vi "Plot Editor.vi"(6 "Original Plot Idx":i32=-1, 7 "Original Graph Name":string, 8 "Error In":errorcluster, 9 "Plot Style in":T2={"Plot Index"=0, "Plot.Bar Plot Style"=0, "Plot.DigitalLineStyle"=1, "Plot.TransitionLocation"=2, "Plot.Transition Type"=0, "Plot.Fill To"=-1, "Plot.Fill/Pt. Color"=16777222, "Plot.Label Format"=3, "Plot.Line Style"=0, "Plot.Line Width"=1, "Plot.Plot Color"=16777222, "Plot.Plot Interpolation"=2, "Plot.Plot Name"="", "Plot.Point Style"=0, "Plot.Visible?"=TRUE, "Plot.XScaleIdx"=0, "Plot.YScaleIdx"=0, "Plot.Anti-aliased"=TRUE}, 10 "Plot in":T3, 11 "Original Graph Refnum":T1) -> (0 "Error Out":errorcluster, 1 "Plot Style out":T2, 2 "Plot out":T3)   [LabVIEW 2021, in "Plot Editor.lvlib"]
uses:
  Plot Editor.lvlib
  XY Graph/XY Graph Plot Properties.ctl
  XY Graph/XY Plot Data.ctl
  XY Graph/XY Graph Refnum.ctl
  Plot Editor Q [Element].ctl
  Plot Editor Q [Event] List.ctl
  Plot Editor Internal Variables.ctl
  XY Graph/XY Graph Event.ctl
  <vilib>/Utility/miscctls.llb/LVPoint32TypeDef.ctl
  <vilib>/Utility/error.llb/DialogType.ctl
  Variant/Variant to Data/Variant to String.vi
  Variant/Variant to Data/Variant to I32.vi
  XY Graph/XY Graph Add-Ons.lvlib
  GUI/GUI.lvlib
  Notebook/Notebook.lvlib
  Graphs.lvlib
  <userlib>/_OpenG.lib/string/string.llb/openg_string.lvlib
  Arrays/Define Ramp Array Dialog.vi
  Arrays/Arrays.lvlib
  Variant/Variant to Data/Variant to Data.lvlib
  Rich Text Box/Rich Text Box.lvlib
  Error/Error.lvlib
  Sound/Sound.lvlib
panel:
  out "Y Array Sum":dbl format="%#_5g"
  out "X Array Sum":dbl format="%#_5g"
  in  "X Array":dbl[](array[numeric])
  in  "Copy":bool
  in  "Cancel":bool
  out "Error":errorcluster
  in  "Reset Style":bool
  out "Y Array Size":i32 format="%#_5g"
  in  "Cancel Data Edit":bool
  in  "OK":bool
  out "X Array Size":i32 format="%#_5g"
  in  "Y Array":dbl[](array[numeric]) caption="X Array"
  out "Plot Preview":cluster{"X Array":dbl[], "Y Array":dbl[]}[](graph)
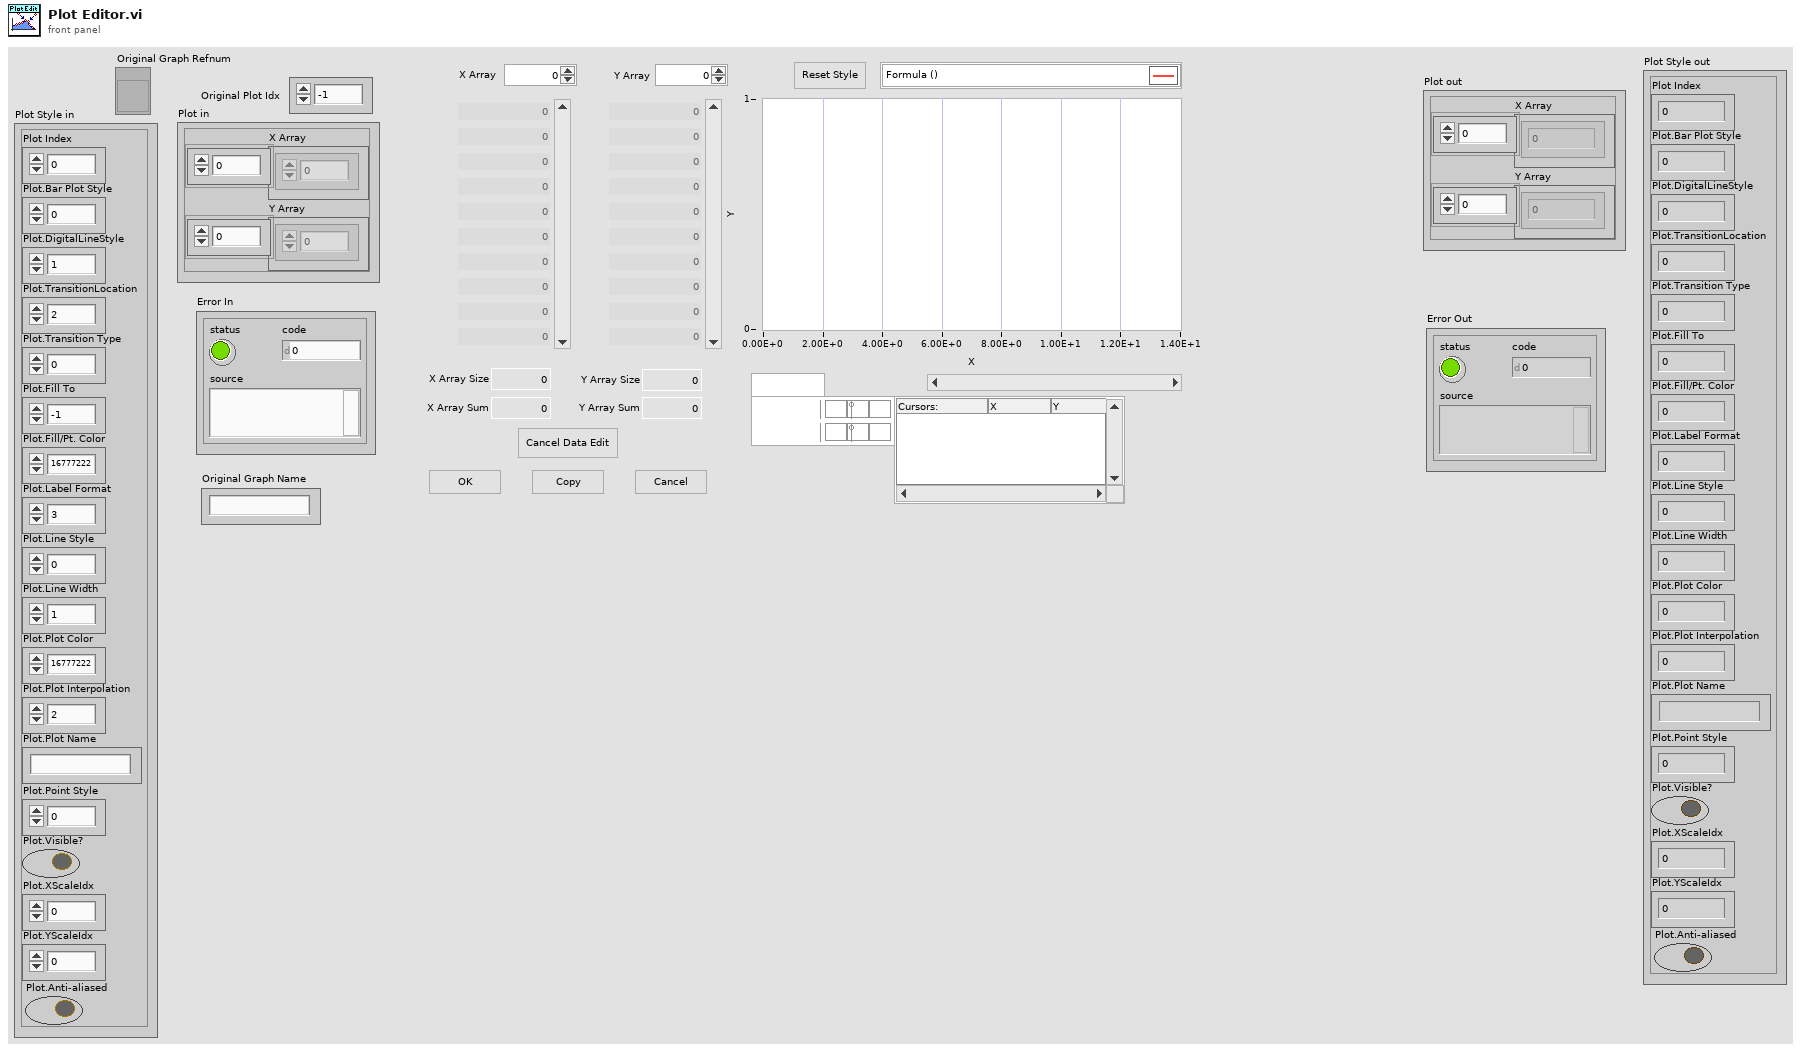
[diagram p1: front panel]
types:
  T1 = typedef "XY Graph Add-Ons.lvlib/XY Graph Refnum.ctl" = refnum<vi>
  T2 = typedef "XY Graph Add-Ons.lvlib/XY Graph Plot Properties.ctl" = cluster{"Plot Index":i32, "Plot.Bar Plot Style":u8, "Plot.DigitalLineStyle":u8, "Plot.TransitionLocation":u8, "Plot.Transition Type":u8, "Plot.Fill To":i16, "Plot.Fill/Pt. Color":u32, "Plot.Label Format":u8, "Plot.Line Style":u8, "Plot.Line Width":u8, "Plot.Plot Color":u32, "Plot.Plot Interpolation":u8, "Plot.Plot Name":string, "Plot.Point Style":u8, "Plot.Visible?":bool, "Plot.XScaleIdx":u32, "Plot.YScaleIdx":u32, "Plot.Anti-aliased":bool}
  T3 = typedef "XY Graph Add-Ons.lvlib/XY Plot Data.ctl" = cluster{"X Array":dbl[], "Y Array":dbl[]}
  T4 = typedef "Plot Editor.lvlib/Plot Editor Q [Element].ctl" = cluster{"Plot Editor Q Event":T5, "Data":variant}
  T5 = typedef "Plot Editor.lvlib/Plot Editor Q [Event] List.ctl" = enum16{"Idle", "Initialization", "Generic XY Graph Event", "Controls >> Store", "Store >> Plot", "Update Plot Style", "Check Data Array Alignment", "Reset Data", "Reset Style", "Accept & Quit", "Copy & Quit", "Save Plot", "Load Plot", "Delete out-of-bound Values", "Delete Element", "Insert Element Before", "Insert Element After", "Update output string", "Delete NaN-containing Pairs", "Delete Pairs with Duplicate X", "Fill Array with Ramp", "Quit"}
  T6 = typedef "Plot Editor.lvlib/Plot Editor Internal Variables.ctl" = cluster{"X Array":dbl[], "Y Array":dbl[], "XY Plot Properties":T2, "X Array Index Values":u32[], "Y Array Index Values":u32[], "Original XY Plot Properties":T2, "Original X Array":dbl[], "Original Y Array":dbl[], "VI title suffix":string, "Refnum based call":bool}
  T7 = typedef "XY Graph Add-Ons.lvlib/XY Graph Event.ctl" = cluster{"Item Tag":string, "XY Graph Refnum":refnum<vi>, "Coords":T8, "Item Path":string}
  T8 = typedef "LVPoint32TypeDef.ctl" = cluster{"Horizontal":i32, "Vertical":i32}
  T9 = typedef "Rich Text Box.lvlib/Text Formatting.ctl" = cluster{"Font":string, "Text Color":T10, "Text Background Color":T10, "Text Style":enum16{"Regular", "Bold", "Italic", "Underline", "Strikeout"}, "Font Size (Points)":dbl, "Text Alignment":i32}
  T10 = typedef "Rich Text Box.lvlib/Text Colors.ctl" = enum16{"Unchanged", "Black", "Blue", "Brown", "Gray", "Green", "Orange", "Pink", "Red", "White"}
  T11 = typedef "DialogType.ctl" = u16
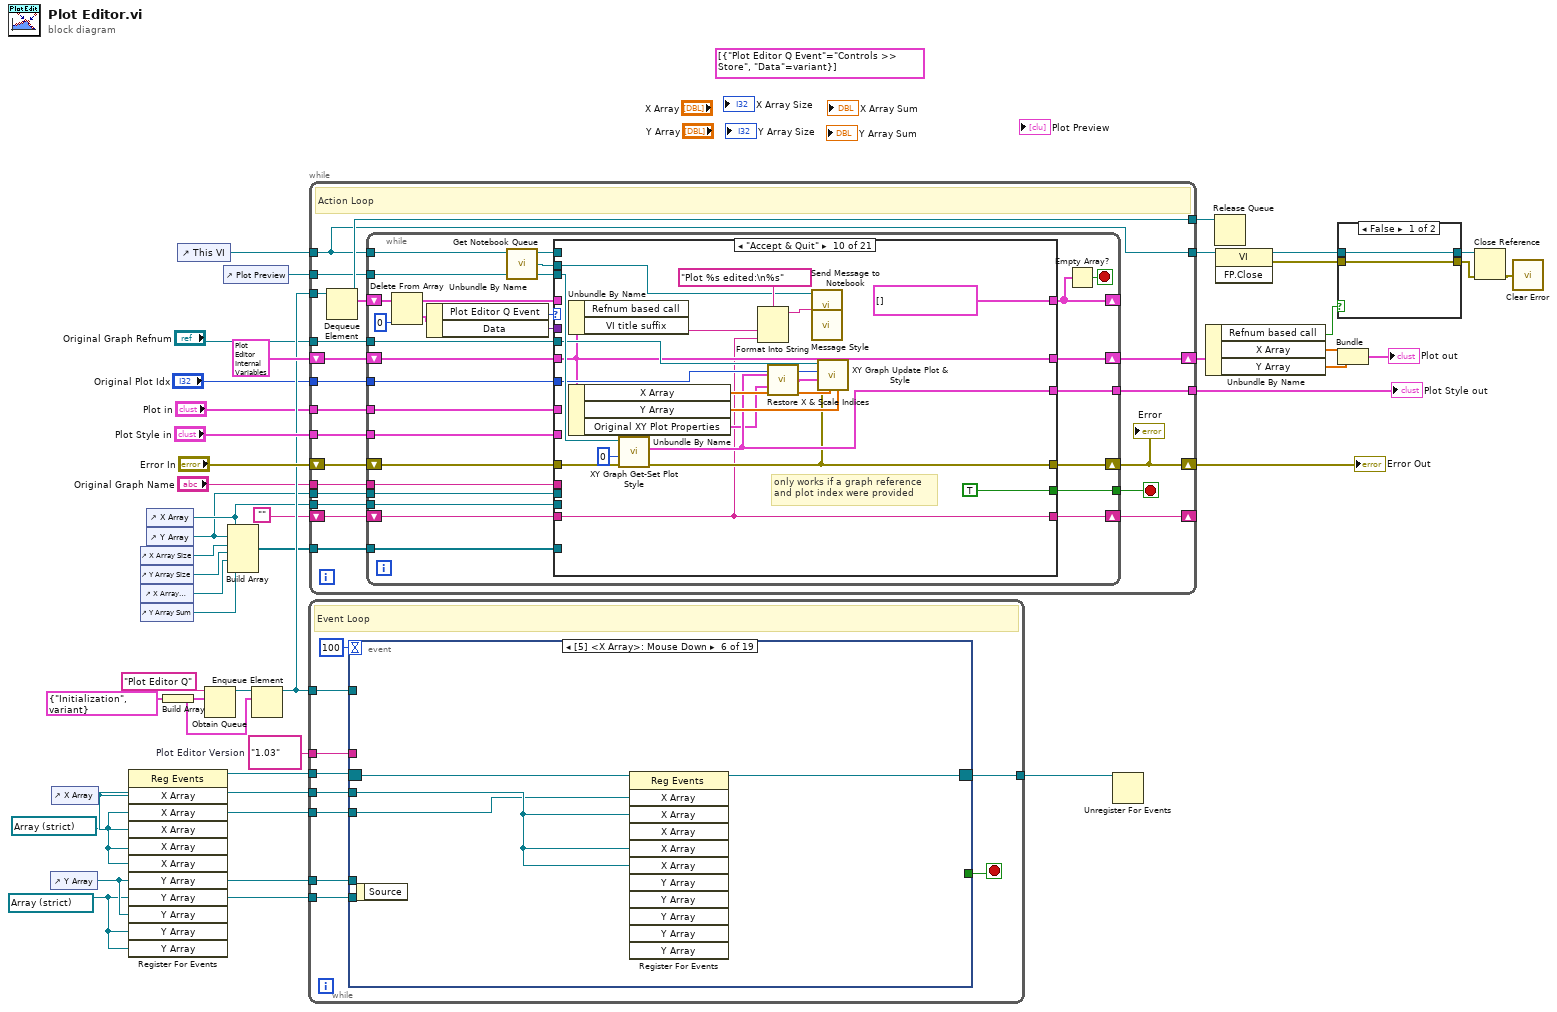
[diagram p0: block diagram]
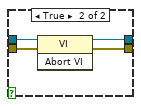
[diagram p2: hidden frame]
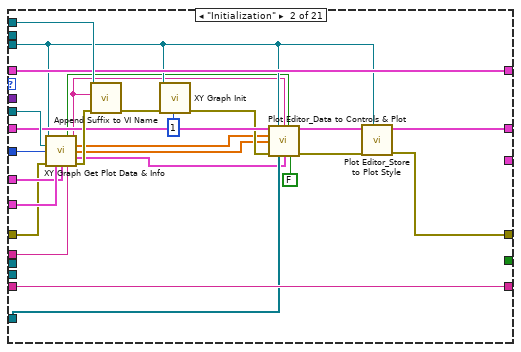
[diagram p4: hidden frame]
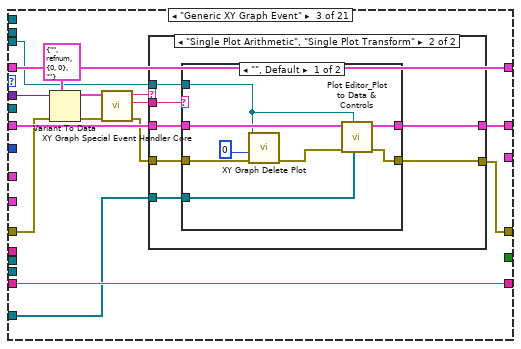
[diagram p5: hidden frame]
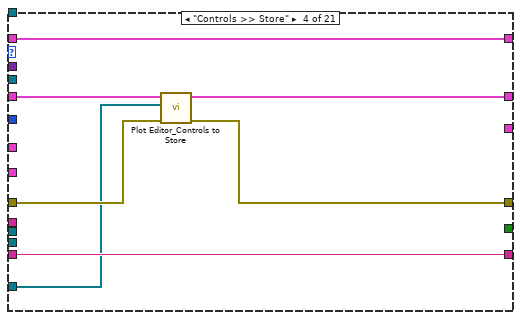
[diagram p8: hidden frame]
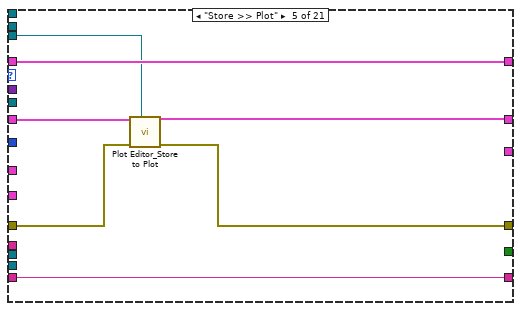
[diagram p9: hidden frame]
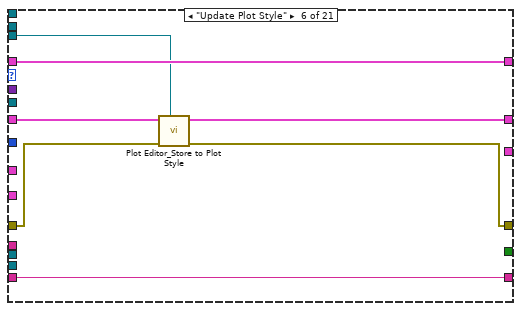
[diagram p10: hidden frame]
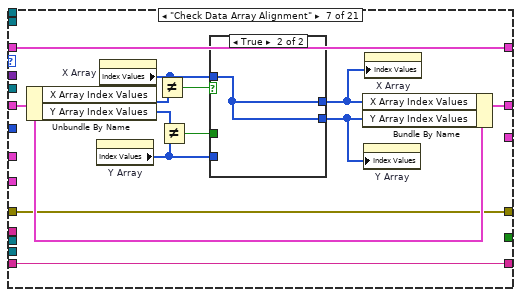
[diagram p11: hidden frame]
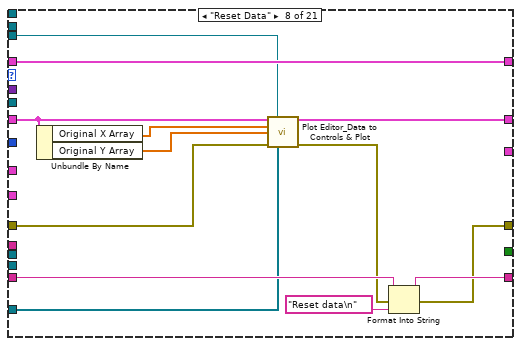
[diagram p14: hidden frame]
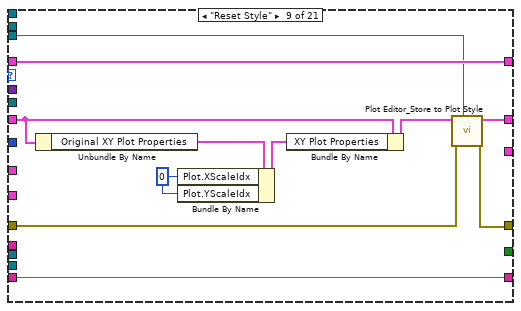
[diagram p15: hidden frame]
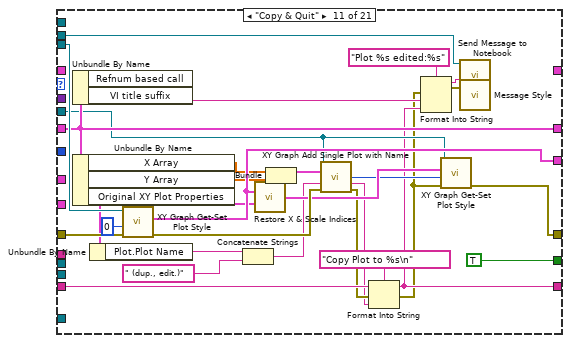
[diagram p16: hidden frame]
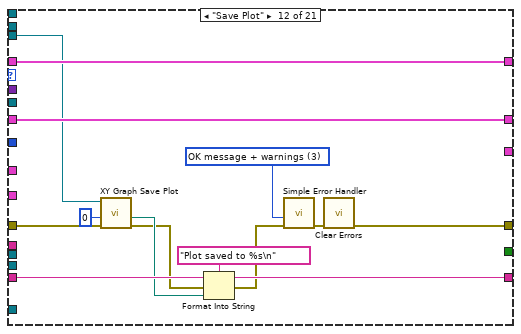
[diagram p17: hidden frame]
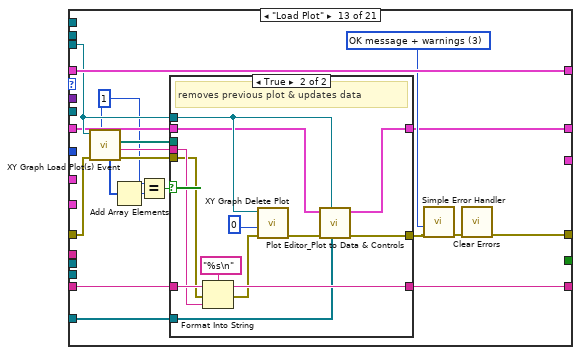
[diagram p18: hidden frame]
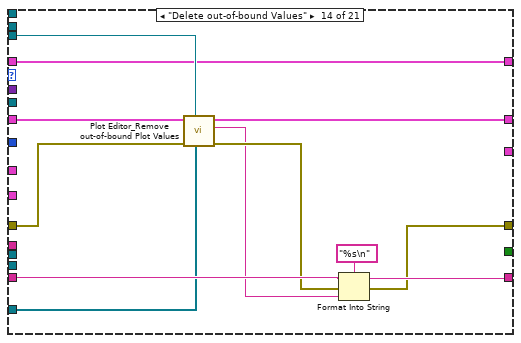
[diagram p20: hidden frame]
diagram:
  w4 = refnum<vi> refnum ("Y Array")
  w3 = refnum<vi> refnum ("X Array")
  (unwired) T4[] [{"Plot Editor Q Event"=enum."Controls >> Store", "Data"=variant}] ("array")
  w27 = "1.03"  # Plot Editor Version
  n1 = control-ref of="Y Array"() -> (w5:refnum<vi>)
  n2 = control-ref of="X Array"() -> (w6:refnum<vi>)
  n3 = register-events(w6, w3, w6, w3, w3, w5, w4, w5, w4, w4) -> (reference out=w26:refnum<event-registration>)  [unwired: 2 in, 1 out]
  n4 = control-ref of="X Array Size"() -> (w9:refnum<vi>)
  n5 = control-ref of="Y Array Size"() -> (w8:refnum<vi>)
  n6 = control-ref of="X Array Sum"() -> (w2:refnum<vi>)
  n7 = control-ref of="Y Array Sum"() -> (w1:refnum<vi>)
  n8 = control-ref of="X Array"() -> (w11:refnum<vi>)
  n9 = control-ref of="Y Array"() -> (w10:refnum<vi>)
  n10 = Build Array(T4 {"Plot Editor Q Event"=enum."Initialization", "Data"=variant} ("Plot Editor Q Element")) -> (w28:T4[])
  n11 = control-ref of="This VI"() -> (w18:refnum<vi>)
  n12 = Obtain Queue(name (unnamed)="Plot Editor Q", element data type=w28) -> (queue out=w41:refnum<queue>)  [unwired: 3 in, 2 out]
  n13 = control-ref of="Plot Preview"() -> (w36:refnum<vi>)
  n14 = Build Array(w11, w10, w9, w8, w2, w1) -> (w7:refnum<vi>[])
  n15 = Enqueue Element(queue=w41, element=w28) -> (queue out=w29:refnum<queue>)  [unwired: 2 in, 2 out]
  n16 = while {
    tunnel: w29 -> [w52]
    tunnel: w27 -> [w51]
    tunnel: w26 -> [w50]
    tunnel: w6 -> [w49]
    tunnel: w5 -> [w48]
    tunnel: [w47] -> w25
    tunnel: w3 -> [w46]
    tunnel: w4 -> [w45]
    stop <- w53 stop-if-true
    # "Event Loop"
    n17 = event shown="[5] <X Array>: Mouse Down" {
      selector: w50 -> [_ _ _ _ _ w179 w183 w186 w189 w195 w201 w205 w210 _ _ _ _ _ _]
      dyn-events: [_ _ _ _ _ w178 w182 w186 w189 w194 w200 w204 w209 _ _ _ _ _ _] -> w47
      timeout: 100 -> [_ _ _ _ _ _ _ _ _ _ _ _ _ _ _ _ _ _ _]
      tunnel: [w56 w58 _ _ _ _ _ _ _ _ _ _ _ _ _ _ TRUE ("Discard?") TRUE ("Discard?") TRUE ("Discard?")] -> w53
      tunnel: w52 -> [w55 w59 w102 w133 w160 _ _ w185 w188 w191 w196 _ _ w220 w222 w224 w227 w230 w233]
      tunnel: w51 -> [_ w57 _ _ _ _ _ _ _ _ _ _ _ _ _ _ _ _ _]
      tunnel: w49 -> [_ _ _ _ _ w177 _ _ _ w193 _ w203 w208 _ _ _ _ _ _]
      tunnel: w48 -> [_ _ _ _ _ _ w181 _ _ _ w198 _ w207 _ _ _ _ _ _]
      tunnel: w46 -> [_ _ _ _ _ w176 _ _ _ w192 _ w202 _ _ _ _ _ _ _]
      tunnel: w45 -> [_ _ _ _ _ _ w180 _ _ _ w199 _ w206 _ _ _ _ _ _]
      event Panel Close? {
        w56 = TRUE ("Discard?")
        n18 = event-data() -> ()  [unwired: 1 in, 1 out]
        n19 = Enqueue Element(queue=w55, element=T4[] [{"Plot Editor Q Event"=enum."Quit", "Data"=variant}]) -> ()  [unwired: 2 in, 3 out]
        n20 = event-data("Discard?"=w56) -> ()  [unwired: 1 in, 1 out]
      }
      event Menu Selection (User) {
        n21 = event-data() -> ("ItemTag"=w60:string)  [unwired: 1 in]
        n22 = case shown="\"Paste Data from Clipboard\"" w60 {
          tunnel: w59 -> [_ w62 w64 w68 w87 _]
          tunnel: [_ _ _ w65 _ _] -> w58
          tunnel: w57 -> [_ _ _ _ _ w95]
          frame "", Default {
          }
          frame "Save Plot" {
            n23 = Enqueue Element(queue=w62, element=T4[] [{"Plot Editor Q Event"=enum."Save Plot", "Data"=variant}]) -> ()  [unwired: 2 in, 3 out]
          }
          frame "Load Plot" {
            n24 = Enqueue Element(queue=w64, element=T4[] [{"Plot Editor Q Event"=enum."Load Plot", "Data"=variant}]) -> ()  [unwired: 2 in, 3 out]
          }
          frame "Quit" {
            n25 = call "Two Buttons Dialog Window with Resizeable Message.vi"("Message"="Are you sure you want to quit Plot Editor?\nQuitting will save the current changes and return to the original graph." ("message"), "OK Button Text"="Accept & Quit" ("T button name (\"OK\")")) -> ("OK?"=w65:bool)  [unwired: 7 in]
            n26 = case shown="True" w65 {
              tunnel: w68 -> [_ w70]
              frame False {
              }
              frame True {
                n27 = Enqueue Element(queue=w70, element=T4[] [{"Plot Editor Q Event"=enum."Accept & Quit", "Data"=variant}]) -> ()  [unwired: 2 in, 3 out]
              }
            }
          }
          frame "Paste Data from Clipboard" {
            w80 = "\n"
            n28 = invoke class="App" method="Clipboard.Read"() -> ("Read Clipbrd"=w76:string)  [unwired: 3 in, 2 out]
            n29 = call <userlib>:"String to 1D Array__ogtk.vi"("delimiter (Tab)"=w80, "string"=w76) -> ("Array of Strings"=w85:string[])  [unwired: 9 in]
            n30 = Delete From Array(array=w85, length=1, index=0) -> (array with subset deleted=w82:string[])  [unwired: 1 out]
            n31 = call <userlib>:"1D Array to String__ogtk.vi"("delimiter (Tab)"=w80, "Array of Strings"=w82) -> ("delimited string"=w81:string)  [unwired: 9 in]
            n32 = Spreadsheet String To Array(format string="%#g", spreadsheet string=w81) -> (array=w88:dbl[][])  [unwired: 2 in]
            n33 = Transpose 2D Array(2D array=w88) -> (transposed array=w79:dbl[][])
            n34 = Index Array(array=w79) -> (element #1=w72:dbl[], element #2=w71:dbl[])  [unwired: 4 in]
            n35 = Array Size(array=w72) -> (size(s)=w78:i32)
            n36 = Array Size(array=w71) -> (size(s)=w77:i32)
            n37 = Empty Array?(array=w72) -> (empty?=w75:bool)
            n38 = Not Equal?(x=w78, y=w77) -> (x != y?=w74:bool)
            n39 = Or(x=w75, y=w74) -> (x .or. y?=w73:bool)
            n40 = case shown="True" w73 {
              tunnel: w87 -> [w92 _]
              tunnel: w72 -> [w90 _]
              tunnel: w71 -> [w89 _]
              frame False {
                n41 = local write "X Array"(w90) -> ()
                n42 = local write "Y Array"(w89) -> ()
                n43 = Enqueue Element(queue=w92, element=T4[] [{"Plot Editor Q Event"=enum."Controls >> Store", "Data"=variant}, {"Plot Editor Q Event"=enum."Store >> Plot", "Data"=variant}]) -> ()  [unwired: 2 in, 3 out]
              }
              frame True {
                n44 = One Button Dialog(message="The clipboard doesn't contain any valid plot data...") -> ()  [unwired: 1 in, 1 out]
                n45 = call "Play Error Sound.vi"() -> ()  [unwired: 27 in, 1 out]
              }
            }
          }
          frame "About..." {
            n46 = Format Into String(format string="                                      Plot Editor\n                                      version %s\n\n                              Author: X. Michalet\n(c) 2017-2022 The Regents of the  University of California" ("message"), w95) -> (resulting string=w94:string)  [unwired: 2 in, 1 out]
            n47 = One Button Dialog(message=w94) -> ()  [unwired: 1 in, 1 out]
          }
        }
      }
      event "X Array": Shortcut Menu Selection (User) {
        n48 = event-data() -> ("ItemTag"=w103:string, "CtlRef"=w100:refnum<vi>, "Coords"=w99:T8)  [unwired: 1 in]
        n49 = case shown="\"Delete NaN-containing Pairs\"" w103 {
          tunnel: [w104 w110 w116 w122 w125 w127] -> w101
          tunnel: w100 -> [_ w109 w115 w121 _ _]
          tunnel: w99 -> [_ w108 w114 w120 _ _]
          frame "", Default {
            n50 = Build Array(T4 {"Plot Editor Q Event"=enum."Idle", "Data"=variant} ("Plot Editor Q Element")) -> (w104:T4[])
          }
          frame "Delete Element" {
            n51 = Bundle("CtlRef"=w109, "Coords"=w108) -> (w106:cluster{"CtlRef":refnum<vi>, "Coords":T8})  [unwired: 1 in]
            n52 = Bundle By Name(cluster=T4 {"Plot Editor Q Event"=enum."Delete Element", "Data"=variant} ("Plot Editor Q Element"), "Data"=w106) -> (w107:T4)
            n53 = Build Array(w107) -> (w110:T4[])
          }
          frame "Insert Element Before" {
            n54 = Bundle("CtlRef"=w115, "Coords"=w114) -> (w112:cluster{"CtlRef":refnum<vi>, "Coords":T8})  [unwired: 1 in]
            n55 = Bundle By Name(cluster=T4 {"Plot Editor Q Event"=enum."Insert Element Before", "Data"=variant} ("Plot Editor Q Element"), "Data"=w112) -> (w113:T4)
            n56 = Build Array(w113) -> (w116:T4[])
          }
          frame "Insert Element After" {
            n57 = Bundle("CtlRef"=w121, "Coords"=w120) -> (w118:cluster{"CtlRef":refnum<vi>, "Coords":T8})  [unwired: 1 in]
            n58 = Bundle By Name(cluster=T4 {"Plot Editor Q Event"=enum."Insert Element After", "Data"=variant} ("Plot Editor Q Element"), "Data"=w118) -> (w119:T4)
            n59 = Build Array(w119) -> (w122:T4[])
          }
          frame "Fill Array with Ramp" {
            n60 = Build Array(T4 {"Plot Editor Q Event"=enum."Fill Array with Ramp", "Data"=variant} ("Plot Editor Q Element")) -> (w125:T4[])
          }
          frame "Delete NaN-containing Pairs" {
            n61 = Build Array(T4 {"Plot Editor Q Event"=enum."Delete NaN-containing Pairs", "Data"=variant} ("Plot Editor Q Element")) -> (w127:T4[])
          }
        }
        n62 = Build Array (concatenate)(w101, T4[] [{"Plot Editor Q Event"=enum."Controls >> Store", "Data"=variant}, {"Plot Editor Q Event"=enum."Store >> Plot", "Data"=variant}] ("array")) -> (w98:T4[])
        n63 = Enqueue Element(queue=w102, element=w98) -> ()  [unwired: 2 in, 3 out]
      }
      event "Y Array": Shortcut Menu Selection (User) {
        n64 = event-data() -> ("ItemTag"=w134:string, "CtlRef"=w132:refnum<vi>, "Coords"=w131:T8)  [unwired: 1 in]
        n65 = case shown="\"Remove NaN-containing Pairs\"" w134 {
          tunnel: [w135 w139 w145 w151 w156] -> w130
          tunnel: w132 -> [_ w138 w144 w150 _]
          tunnel: w131 -> [_ w137 w143 w149 _]
          frame "", Default {
            n66 = Build Array(T4 {"Plot Editor Q Event"=enum."Idle", "Data"=variant} ("Plot Editor Q Element")) -> (w135:T4[])
          }
          frame "Delete Element" {
            n67 = Bundle("CtlRef"=w138, "Coords"=w137) -> (w141:cluster{"CtlRef":refnum<vi>, "Coords":T8})  [unwired: 1 in]
            n68 = Bundle By Name(cluster=T4 {"Plot Editor Q Event"=enum."Delete Element", "Data"=variant} ("Plot Editor Q Element"), "Data"=w141) -> (w142:T4)
            n69 = Build Array(w142) -> (w139:T4[])
          }
          frame "Insert Element Before" {
            n70 = Bundle("CtlRef"=w144, "Coords"=w143) -> (w147:cluster{"CtlRef":refnum<vi>, "Coords":T8})  [unwired: 1 in]
            n71 = Bundle By Name(cluster=T4 {"Plot Editor Q Event"=enum."Insert Element Before", "Data"=variant} ("Plot Editor Q Element"), "Data"=w147) -> (w148:T4)
            n72 = Build Array(w148) -> (w145:T4[])
          }
          frame "Insert Element After" {
            n73 = Bundle("CtlRef"=w150, "Coords"=w149) -> (w153:cluster{"CtlRef":refnum<vi>, "Coords":T8})  [unwired: 1 in]
            n74 = Bundle By Name(cluster=T4 {"Plot Editor Q Event"=enum."Insert Element After", "Data"=variant} ("Plot Editor Q Element"), "Data"=w153) -> (w154:T4)
            n75 = Build Array(w154) -> (w151:T4[])
          }
          frame "Remove NaN-containing Pairs" {
            n76 = Build Array(T4 {"Plot Editor Q Event"=enum."Delete NaN-containing Pairs", "Data"=variant} ("Plot Editor Q Element")) -> (w156:T4[])
          }
        }
        n77 = Build Array (concatenate)(w130, T4[] [{"Plot Editor Q Event"=enum."Controls >> Store", "Data"=variant}, {"Plot Editor Q Event"=enum."Store >> Plot", "Data"=variant}] ("array")) -> (w129:T4[])
        n78 = Enqueue Element(queue=w133, element=w129) -> ()  [unwired: 2 in, 3 out]
      }
      event "Plot Preview": Shortcut Menu Selection (User) {
        n79 = event-data() -> ("ItemTag"=w161:string, "CtlRef"=w159:refnum<vi>, "Coords"=w158:T8, "ItemPath"=w157:string)  [unwired: 1 in]
        n80 = case shown="\"Load Plot\"" w161 {
          selector: w161 -> [w170 _ _]
          tunnel: w160 -> [w166 w173 w175]
          tunnel: w159 -> [w169 _ _]
          tunnel: w158 -> [w168 _ _]
          tunnel: w157 -> [w167 _ _]
          frame "", Default {
            n81 = Bundle By Name(cluster=T7 {"Item Tag"="", "XY Graph Refnum"=refnum, "Coords"={"Horizontal"=0, "Vertical"=0}, "Item Path"=""} ("XY Graph Event"), "Item Tag"=w170, "XY Graph Refnum"=w169, "Coords"=w168, "Item Path"=w167) -> (w163:T7)
            n82 = Bundle By Name(cluster=T4 {"Plot Editor Q Event"=enum."Generic XY Graph Event", "Data"=variant} ("element"), "Data"=w163) -> (w164:T4)
            n83 = Build Array(w164) -> (w162:T4[])
            n84 = Enqueue Element(queue=w166, element=w162) -> ()  [unwired: 2 in, 3 out]
          }
          frame "Load Plot" {
            n85 = Enqueue Element(queue=w173, element=T4[] [{"Plot Editor Q Event"=enum."Load Plot", "Data"=variant}]) -> ()  [unwired: 2 in, 3 out]
          }
          frame "Delete out-of-bound Values" {
            n86 = Enqueue Element(queue=w175, element=T4[] [{"Plot Editor Q Event"=enum."Delete out-of-bound Values", "Data"=variant}]) -> ()  [unwired: 2 in, 3 out]
          }
        }
      }
      event Mouse Down {
        n87 = event-data() -> ()  [unwired: 1 in, 1 out]
        n88 = register-events(reference=w179, w176, w177, w177, w177) -> (reference out=w178:refnum<event-registration>)  [unwired: 7 in, 1 out]
      }
      event Mouse Down {
        n89 = event-data() -> ()  [unwired: 1 in, 1 out]
        n90 = register-events(reference=w183, w180, w181, w181, w181) -> (reference out=w182:refnum<event-registration>)  [unwired: 7 in, 1 out]
      }
      event Mouse Move; Mouse Wheel {
        n91 = event-data() -> ()  [unwired: 1 in, 1 out]
        n92 = Enqueue Element(queue=w185, element=T4[] [{"Plot Editor Q Event"=enum."Check Data Array Alignment", "Data"=variant}]) -> ()  [unwired: 2 in, 3 out]
      }
      event Timeout {
        n93 = event-data() -> ()  [unwired: 1 in, 1 out]
        n94 = Enqueue Element(queue=w188, element=T4[] [{"Plot Editor Q Event"=enum."Check Data Array Alignment", "Data"=variant}]) -> ()  [unwired: 2 in, 3 out]
      }
      event Mouse Up {
        n95 = event-data() -> ()  [unwired: 1 in, 1 out]
        n96 = register-events(reference=w195, w193, w192, w192) -> (reference out=w194:refnum<event-registration>)  [unwired: 8 in, 1 out]
        n97 = Enqueue Element(queue=w191, element=T4[] [{"Plot Editor Q Event"=enum."Check Data Array Alignment", "Data"=variant}]) -> ()  [unwired: 2 in, 3 out]
      }
      event Mouse Up {
        n98 = event-data() -> ()  [unwired: 1 in, 1 out]
        n99 = register-events(reference=w201, w198, w199, w199) -> (reference out=w200:refnum<event-registration>)  [unwired: 8 in, 1 out]
        n100 = Enqueue Element(queue=w196, element=T4[] [{"Plot Editor Q Event"=enum."Check Data Array Alignment", "Data"=variant}]) -> ()  [unwired: 2 in, 3 out]
      }
      event Mouse Leave {
        n101 = event-data() -> ()  [unwired: 1 in, 1 out]
        n102 = register-events(reference=w205, w203, w202, w202, w202) -> (reference out=w204:refnum<event-registration>)  [unwired: 7 in, 1 out]
      }
      event Mouse Leave {
        n103 = event-data() -> ()  [unwired: 1 in, 1 out]
        n104 = register-events(reference=w210, w208, w207, w206, w206, w206) -> (reference out=w209:refnum<event-registration>)  [unwired: 6 in, 1 out]
      }
      event "X Array", "Y Array": Value Change {
        n105 = event-data() -> ("CtlRef"=w215:refnum<vi>)  [unwired: 1 in]
        n106 = property class="Arr (strict)"(reference=w215) -> (error out=w212:errorcluster, "Label.Text"=w213:string)  [unwired: 1 in, 1 out]
        n107 = Format Into String(format string="User added %s data", error in=w212, w213) -> (resulting string=w211:string)  [unwired: 1 in, 1 out]
        n108 = Bundle By Name(cluster=T4 {"Plot Editor Q Event"=enum."Update output string", "Data"=variant} ("Plot Editor Q Element"), "Data"=w211) -> (w216:T4)
        n109 = Build Array (concatenate)(T4[] [{"Plot Editor Q Event"=enum."Controls >> Store", "Data"=variant}, {"Plot Editor Q Event"=enum."Store >> Plot", "Data"=variant}, {"Plot Editor Q Event"=enum."Check Data Array Alignment", "Data"=variant}] ("element"), w216) -> (w218:T4[])
        n110 = Enqueue Element(queue=w220, element=w218) -> ()  [unwired: 2 in, 3 out]
      }
      event "Reset Style": Value Change {
        n111 = event-data() -> ()  [unwired: 1 in, 1 out]
        n112 = Enqueue Element(queue=w222, element=T4[] [{"Plot Editor Q Event"=enum."Reset Style", "Data"=variant}]) -> ()  [unwired: 2 in, 3 out]
      }
      event "Cancel Data Edit": Value Change {
        n113 = event-data() -> ()  [unwired: 1 in, 1 out]
        n114 = Enqueue Element(queue=w224, element=T4[] [{"Plot Editor Q Event"=enum."Reset Data", "Data"=variant}]) -> ()  [unwired: 2 in, 3 out]
      }
      event "OK": Value Change {
        n115 = event-data() -> ()  [unwired: 1 in, 1 out]
        n116 = Enqueue Element(queue=w227, element=T4[] [{"Plot Editor Q Event"=enum."Accept & Quit", "Data"=variant}]) -> ()  [unwired: 2 in, 3 out]
      }
      event "Copy": Value Change {
        n117 = event-data() -> ()  [unwired: 1 in, 1 out]
        n118 = Enqueue Element(queue=w230, element=T4[] [{"Plot Editor Q Event"=enum."Copy & Quit", "Data"=variant}]) -> ()  [unwired: 2 in, 3 out]
      }
      event "Cancel": Value Change {
        n119 = event-data() -> ()  [unwired: 1 in, 1 out]
        n120 = Enqueue Element(queue=w233, element=T4[] [{"Plot Editor Q Event"=enum."Quit", "Data"=variant}]) -> ()  [unwired: 2 in, 3 out]
      }
    }
  }
  n121 = while {
    tunnel: w29 -> [w254]
    tunnel: [w251] -> w40
    shift-right: [w248] -> w34
    shift-left: T6 {"X Array"=[], "Y Array"=[], "XY Plot Properties"={"Plot Index"=0, "Plot.Bar Plot Style"=0, "Plot.DigitalLineStyle"=0, "Plot.TransitionLocation"=0, "Plot.Transition Type"=0, "Plot.Fill To"=-1, "Plot.Fill/Pt. Color"=0, "Plot.Label Format"=0, "Plot.Line Style"=0, "Plot.Line Width"=0, "Plot.Plot Color"=0, "Plot.Plot Interpolation"=0, "Plot.Plot Name"="Plot", "Plot.Point Style"=0, "Plot.Visible?"=FALSE, "Plot.XScaleIdx"=0, "Plot.YScaleIdx"=0, "Plot.Anti-aliased"=FALSE}, "X Array Index Values"=[], "Y Array Index Values"=[], "Original XY Plot Properties"={"Plot Index"=0, "Plot.Bar Plot Style"=0, "Plot.DigitalLineStyle"=0, "Plot.TransitionLocation"=0, "Plot.Transition Type"=0, "Plot.Fill To"=0, "Plot.Fill/Pt. Color"=0, "Plot.Label Format"=0, "Plot.Line Style"=0, "Plot.Line Width"=0, "Plot.Plot Color"=0, "Plot.Plot Interpolation"=0, "Plot.Plot Name"="", "Plot.Point Style"=0, "Plot.Visible?"=FALSE, "Plot.XScaleIdx"=0, "Plot.YScaleIdx"=0, "Plot.Anti-aliased"=FALSE}, "Original X Array"=[], "Original Y Array"=[], "VI title suffix"="", "Refnum based call"=FALSE} ("Plot Editor Internal Data") -> [w250]
    shift-right: [w239] -> w35
    shift-left: "Error In" -> [w247]
    tunnel: "Plot Style in" -> [w249]
    tunnel: w36 -> [w246]
    tunnel: [w245] -> w30
    tunnel: "Original Graph Refnum" -> [w244]
    tunnel: "Original Plot Idx" -> [w243]
    tunnel: "Plot in" -> [w242]
    tunnel: "Original Graph Name" -> [w241]
    tunnel: w18 -> [w240]
    tunnel: [w240] -> w20
    shift-right: [w237] -> _
    shift-left: "" -> [w238]
    tunnel: w11 -> [w236]
    tunnel: w10 -> [w235]
    tunnel: w7 -> [w234]
    stop <- w252 stop-if-true
    # "Action Loop"
    n122 = Dequeue Element(queue=w254) -> (queue out=w251:refnum<queue>, element=w253:T4[])  [unwired: 2 in, 2 out]
    n123 = while {
      tunnel: [w281] -> w252
      shift-right: [w277] -> _
      shift-left: w253 -> [w280]
      tunnel: w249 -> [w274]
      tunnel: w246 -> [w256]
      shift-right: [w273] -> w248
      shift-left: w250 -> [w275]
      shift-right: [w269] -> w239
      shift-left: w247 -> [w270]
      tunnel: [w268] -> w245
      tunnel: w244 -> [w267]
      tunnel: w243 -> [w266]
      tunnel: w242 -> [w265]
      tunnel: w241 -> [w264]
      tunnel: w240 -> [w263]
      shift-right: [w260] -> w237
      shift-left: w238 -> [w261]
      tunnel: w236 -> [w259]
      tunnel: w235 -> [w258]
      tunnel: w234 -> [w257]
      stop <- w276 stop-if-true
      n124 = Delete From Array(array=w280, index=0) -> (deleted portion=w272:T4, array with subset deleted=w278:T4[])  [unwired: 1 in]
      n125 = Unbundle By Name(w272) -> ("Plot Editor Q Event"=w271:T5, "Data"=w262:variant)
      n126 = call "Get Notebook Queue.vi"() -> ("Notebook Queue"=w255:refnum<queue>)  [unwired: 9 in]
      n127 = case shown="\"Accept & Quit\"" w271 {
        tunnel: [_ _ _ _ _ _ _ _ _ TRUE TRUE _ _ _ _ _ _ _ _ _ TRUE] -> w281
        tunnel: w278 -> [w285 w300 w326 w352 w359 w366 w373 w398 w412 _ _ w476 w495 w515 w531 w576 w621 w668 w673 w706 _]
        tunnel: [w285 w300 w326 w352 w359 w366 w373 w398 w412 T4[] [] _ w476 w495 w515 w530 w575 w620 w668 w673 w703 T4[] []] -> w277
        tunnel: w275 -> [w283 w297 w320 w350 w355 w362 w375 w395 w411 w425 w460 w475 w485 w514 w527 w572 w617 w660 w672 w713 w742]
        tunnel: w274 -> [_ w309 _ _ _ _ _ _ _ _ _ _ _ _ _ _ _ _ _ _ _]
        tunnel: [w283 w298 w319 w349 w356 w361 w374 w394 w405 w425 w460 w475 w484 w513 w524 w571 w616 w660 w670 w712 w743] -> w273
        tunnel: w270 -> [w284 w307 w316 w347 w353 w365 w370 w393 w404 w423 w458 w473 w494 w523 w528 w574 w619 w662 w678 w711 _]
        tunnel: [w284 w299 w317 w348 w354 w364 w370 w397 w403 w421 w454 w470 w491 w518 w529 w573 w618 w663 w676 w704 _] -> w269
        tunnel: [_ _ _ _ _ _ _ _ _ w422 w457 _ _ _ _ _ _ _ _ _ w739] -> w268
        tunnel: w267 -> [_ w311 _ _ _ _ _ _ _ w429 w453 _ _ _ _ _ _ _ _ _ _]
        tunnel: w266 -> [_ w310 _ _ _ _ _ _ _ w428 _ _ _ _ _ _ _ _ _ _ _]
        tunnel: w265 -> [_ w308 _ _ _ _ _ _ _ _ _ _ _ _ _ _ _ _ _ _ _]
        tunnel: w264 -> [_ w306 _ _ _ _ _ _ _ _ _ _ _ _ _ _ _ _ _ _ _]
        tunnel: w263 -> [_ w305 _ _ _ _ _ _ _ _ _ _ _ _ _ _ _ _ _ _ _]
        tunnel: w262 -> [_ _ w321 _ _ _ _ _ _ _ _ _ _ _ w543 w588 w633 w667 w684 _ _]
        tunnel: w259 -> [_ _ _ _ _ _ _ _ _ _ _ _ _ _ w537 w582 w630 _ _ _ _]
        tunnel: w258 -> [_ _ _ _ _ _ _ _ _ _ _ _ _ _ w536 w581 w629 _ _ _ _]
        tunnel: w261 -> [w282 w302 w325 w351 w358 w363 w369 w401 w407 w414 w443 w468 w483 w522 w533 w578 w623 w666 w680 w708 w737]
        tunnel: [w282 w302 w325 w351 w358 w363 w369 w400 w407 w414 w437 w465 w482 w521 w532 w577 w622 w665 w679 w707 w737] -> w260
        tunnel: w257 -> [_ w292 w313 w346 _ _ _ w389 _ _ _ _ w479 w512 w526 w569 w615 _ w671 w702 _]
        tunnel: w256 -> [_ w295 w314 _ w357 w360 _ w390 w402 w431 w462 w474 w487 w517 w525 w570 w614 _ w669 w701 _]
        tunnel: w255 -> [_ _ _ _ _ _ _ _ _ w413 w433 _ _ _ _ _ _ _ _ _ _]
        frame "Idle" {
        }
        frame "Initialization" {
          n128 = call "XY Graph Get Plot Data & Info.vi"("Destination Graph"=w295, "Original Graph"=w311, "Original Plot Idx"=w310, "Error In"=w307, "Plot Style in"=w309, "Plot in"=w308, "Graph Origin Name"=w306) -> ("Refnum based call"=w286:bool, "VI Title Suffix"=w287:string, "X Array"=w291:dbl[], "Y Array"=w290:dbl[], "Plot Style out"=w288:T2, "Error Out"=w304:errorcluster)  [unwired: 3 in]
          n129 = call "Append Suffix to VI Name.vi"("error in (no error)"=w304, "VI Title Suffix"=w287, "VI in"=w305) -> ("Error Out"=w301:errorcluster)  [unwired: 8 in]
          n130 = call "XY Graph Init.vi"("Max Legend Size (8)"=1 ("Plot.XScaleIdx"), "Error In"=w301, "XYGraph in"=w295) -> ("Error Out"=w294:errorcluster)  [unwired: 8 in]
          n131 = call "Plot Editor_Data to Controls & Plot.vi"("Plot Editor Internal Data"=w297, "XYGraph in"=w295, "VI Title Suffix"=w287, "Refnum based call"=w286, "X Array"=w291, "Y Array"=w290, "error in (no error)"=w294, "Control Refnums"=w292, "Plot Style"=w288, "Data only (T)"=FALSE) -> ("Plot Editor Internal Data"=w296:T6, "error out"=w293:errorcluster)  [unwired: 4 in]
          n132 = call "Plot Editor_Store to Plot Style.vi"("XYGraph in"=w295, "error in (no error)"=w293, "Plot Editor Internal Data"=w296) -> ("error out"=w299:errorcluster, "Plot Editor Internal Data (dup)"=w298:T6)  [unwired: 7 in]
        }
        frame "Generic XY Graph Event" {
          n133 = Variant To Data(error in=w316, type=T7 {"Item Tag"="", "XY Graph Refnum"=refnum, "Coords"={"Horizontal"=0, "Vertical"=0}, "Item Path"=""} ("XY Graph Event"), Variant=w321) -> (data=w322:T7, error out=w323:errorcluster)
          n134 = call "XY Graph Special Event Handler Core.vi"("error in (no error)"=w323, "XY Graph Event"=w322) -> ("error out"=w318:errorcluster, "Message"=w312:string, "Menu Item Tag (dup)"=w315:string)  [unwired: 5 in, 2 out]
          n135 = case shown="\"Single Plot Arithmetic\", \"Single Plot Transform\"" w315 {
            tunnel: w320 -> [w328 w335]
            tunnel: [w328 w332] -> w319
            tunnel: w318 -> [w327 w334]
            tunnel: [w327 w331] -> w317
            tunnel: w314 -> [_ w333]
            tunnel: w313 -> [_ w330]
            tunnel: w312 -> [_ w329]
            frame "", Default {
            }
            frame "Single Plot Arithmetic", "Single Plot Transform" {
              n136 = case shown="\"\", Default" w329 {
                tunnel: w335 -> [w342 w345]
                tunnel: w334 -> [w341 w344]
                tunnel: w333 -> [w339 _]
                tunnel: [w338 w345] -> w332
                tunnel: [w337 w344] -> w331
                tunnel: w330 -> [w336 _]
                frame "", Default {
                  n137 = call "XY Graph Delete Plot.vi"("Error In"=w341, "Plot Index"=0, "XYGraph Ref"=w339) -> ("Error Out"=w340:errorcluster)  [unwired: 5 in, 3 out]
                  n138 = call "Plot Editor_Plot to Data & Controls.vi"("Control Refnums"=w336, "XYGraph in"=w339, "error in (no error)"=w340, "Plot Editor Internal Data in"=w342) -> ("error out"=w337:errorcluster, "Plot Editor Internal Data out"=w338:T6)  [unwired: 6 in]
                }
                frame "Operation cancelled by user." {
                }
              }
            }
          }
        }
        frame "Controls >> Store" {
          n139 = call "Plot Editor_Controls to Store.vi"("Error In"=w347, "Control Refnums"=w346, "Plot Editor Internal Data in"=w350) -> ("Error Out"=w348:errorcluster, "Plot Editor Internal Data out"=w349:T6)  [unwired: 7 in]
        }
        frame "Store >> Plot" {
          n140 = call "Plot Editor_Store to Plot.vi"("XYGraph in"=w357, "Error In"=w353, "Plot Editor Internal Data"=w355) -> ("Error Out"=w354:errorcluster, "Plot Editor Internal Data (dup)"=w356:T6)  [unwired: 7 in]
        }
        frame "Update Plot Style" {
          n141 = call "Plot Editor_Store to Plot Style.vi"("XYGraph in"=w360, "error in (no error)"=w365, "Plot Editor Internal Data"=w362) -> ("error out"=w364:errorcluster, "Plot Editor Internal Data (dup)"=w361:T6)  [unwired: 7 in]
        }
        frame "Check Data Array Alignment" {
          n142 = Unbundle By Name(w375) -> ("X Array Index Values"=w379:u32[], "Y Array Index Values"=w378:u32[])
          n143 = property on="Y Array" class="Arr (strict)"() -> ("Index Values"=w371:u32[])  [unwired: 2 in, 2 out]
          n144 = property on="X Array" class="Arr (strict)"() -> ("Index Values"=w376:u32[])  [unwired: 2 in, 2 out]
          n145 = Not Equal?(x=w376, y=w379) -> (x != y?=w377:bool)
          n146 = Not Equal?(x=w378, y=w371) -> (x != y?=w372:bool)
          n147 = case shown="True" w377 {
            tunnel: w376 -> [w380 w388]
            tunnel: [w381 w388] -> w367
            tunnel: [w382 w388] -> w368
            tunnel: w372 -> [w384 _]
            tunnel: w371 -> [w383 _]
            frame False {
              n148 = case shown="False" w384 {
                tunnel: w383 -> [w385 w387]
                tunnel: [w386 w387] -> w382
                tunnel: [w385 w387] -> w381
                tunnel: w380 -> [w386 _]
                frame False {
                }
                frame True {
                }
              }
            }
            frame True {
            }
          }
          n149 = Bundle By Name(cluster=w375, "X Array Index Values"=w368, "Y Array Index Values"=w367) -> (w374:T6)
          n150 = property on="Y Array" class="Arr (strict)"("Index Values"=w367) -> ()  [unwired: 2 in, 2 out]
          n151 = property on="X Array" class="Arr (strict)"("Index Values"=w368) -> ()  [unwired: 2 in, 2 out]
        }
        frame "Reset Data" {
          n152 = Unbundle By Name(w395) -> ("Original X Array"=w396:dbl[], "Original Y Array"=w392:dbl[])
          n153 = call "Plot Editor_Data to Controls & Plot.vi"("Plot Editor Internal Data"=w395, "XYGraph in"=w390, "X Array"=w396, "Y Array"=w392, "error in (no error)"=w393, "Control Refnums"=w389) -> ("Plot Editor Internal Data"=w394:T6, "error out"=w391:errorcluster)  [unwired: 8 in]
          n154 = Format Into String(initial string=w401, error in=w391, "Reset data\n" ("format string")) -> (resulting string=w400:string, error out=w397:errorcluster)  [unwired: 1 in]
        }
        frame "Reset Style" {
          w408 = u32 0 ("Plot.XScaleIdx")
          n155 = Unbundle By Name(w411) -> ("Original XY Plot Properties"=w410:T2)
          n156 = Bundle By Name(cluster=w410, "Plot.XScaleIdx"=w408, "Plot.YScaleIdx"=w408) -> (w409:T2)
          n157 = Bundle By Name(cluster=w411, "XY Plot Properties"=w409) -> (w406:T6)
          n158 = call "Plot Editor_Store to Plot Style.vi"("XYGraph in"=w402, "error in (no error)"=w404, "Plot Editor Internal Data"=w406) -> ("error out"=w403:errorcluster, "Plot Editor Internal Data (dup)"=w405:T6)  [unwired: 7 in]
        }
        frame "Accept & Quit" {
          # "only works if a graph reference\nand plot index were provided"
          n159 = Unbundle By Name(w425) -> ("VI title suffix"=w424:string)  [unwired: 1 out]
          n160 = Unbundle By Name(w425) -> ("X Array"=w427:dbl[], "Y Array"=w426:dbl[], "Original XY Plot Properties"=w418:T2)
          n161 = call "XY Graph Get-Set Plot Style.vi"("Error In"=w423, "Plot Index"=0, "XYGraph in"=w431) -> ("Error Out"=w421:errorcluster, "Plot Style out"=w422:T2)  [unwired: 5 in, 2 out]
          n162 = Format Into String(format string="Plot %s edited:\n%s", w424, w414) -> (resulting string=w415:string)  [unwired: 2 in, 1 out]
          n163 = call "Restore X & Scale Indices.vi"("New Plot Style in"=w422, "Original Plot Style in"=w418) -> ("Updated Plot Style out"=w419:T2)  [unwired: 13 in]
          n164 = call "Message Style.vi"() -> ("Message Formatting"=w416:T9)
          n165 = call "Send Message to Notebook.vi"("Text Formatting"=w416, "Message"=w415, "Notebook Queue"=w413) -> ()  [unwired: 5 in, 2 out]
          n166 = call "XY Graph Update Plot & Style.vi"("Y Array"=w426, "X Array"=w427, "Error In"=w421, "XY Plot Style in"=w419, "Plot Idx"=w428, "XY Graph refnum"=w429) -> ()  [unwired: 3 in, 3 out]
        }
        frame "Copy & Quit" {
          n167 = Unbundle By Name(w460) -> ("VI title suffix"=w459:string)  [unwired: 1 out]
          n168 = Unbundle By Name(w460) -> ("X Array"=w448:dbl[], "Y Array"=w447:dbl[], "Original XY Plot Properties"=w445:T2)
          n169 = Unbundle By Name(w445) -> ("Plot.Plot Name"=w444:string)
          n170 = call "XY Graph Get-Set Plot Style.vi"("Error In"=w458, "Plot Index"=0, "XYGraph in"=w462) -> ("Error Out"=w455:errorcluster, "Plot Style out"=w457:T2)  [unwired: 5 in, 2 out]
          n171 = Concatenate Strings(w444, " (dup., edit.)" ("string")) -> (w449:string)
          n172 = call "Restore X & Scale Indices.vi"("New Plot Style in"=w457, "Original Plot Style in"=w445) -> ("Updated Plot Style out"=w452:T2)  [unwired: 13 in]
          n173 = Bundle("X Array"=w448, "Y Array"=w447) -> (w446:cluster{"X Array":dbl[], "Y Array":dbl[]})  [unwired: 1 in]
          n174 = call "XY Graph Add Single Plot with Name.vi"("XYGraph Ref in"=w453, "Plot"=w446, "Plot Name (\"Plot\")"=w449, "error in (no error)"=w455) -> ("Plot Index"=w451:i32, "Plot Name"=w438:string, "error out"=w440:errorcluster)  [unwired: 8 in, 1 out]
          n175 = Format Into String(format string="Copy Plot to %s\n", initial string=w443, error in=w440, w438) -> (resulting string=w437:string, error out=w435:errorcluster)
          n176 = Format Into String(format string="Plot %s edited:%s", error in=w435, w459, w437) -> (resulting string=w441:string, error out=w434:errorcluster)  [unwired: 1 in]
          n177 = call "XY Graph Get-Set Plot Style.vi"("Error In"=w435, "Plot Index"=w451, "Plot Style in"=w452, "XYGraph in"=w453) -> ("Error Out"=w454:errorcluster)  [unwired: 4 in, 3 out]
          n178 = call "Message Style.vi"() -> ("Message Formatting"=w442:T9)
          n179 = call "Send Message to Notebook.vi"("Text Formatting"=w442, "Error In"=w434, "Message"=w441, "Notebook Queue"=w433) -> ()  [unwired: 4 in, 2 out]
        }
        frame "Save Plot" {
          w471 = T11 3 items=["no dialog", "OK message", "continue or stop message", "OK message + warnings", "continue/stop + warnings"] ("type of dialog (OK msg:1)")
          n180 = call "XY Graph Save Plot.vi"("Error In"=w473, "Plot Index (-1: last plot)"=0 ("Plot Index"), "XYGraph Ref"=w474) -> ("Error Out"=w464:errorcluster, "File Path"=w466:path)  [unwired: 3 in, 4 out]
          n181 = Format Into String(format string="Plot saved to %s\n", initial string=w468, error in=w464, w466) -> (resulting string=w465:string, error out=w463:errorcluster)
          n182 = call <vilib>:"Simple Error Handler.vi"("type of dialog (OK msg:1)"=w471, "error in (no error)"=w463) -> ("error out"=w472:errorcluster)  [unwired: 3 in, 4 out]
          n183 = call <vilib>:"Clear Errors.vi"("error in (no error)"=w472) -> ("error out"=w470:errorcluster)  [unwired: 5 in, 1 out]
        }
        frame "Load Plot" {
          w492 = T11 3 items=["no dialog", "OK message", "continue or stop message", "OK message + warnings", "continue/stop + warnings"] ("type of dialog (OK msg:1)")
          w477 = 1 ("Max Number of Plot to Load (-1: All)")
          n184 = call "XY Graph Load Plot(s) Event.vi"("Max Number of Plot to Load (-1: All)"=w477, "Error In"=w494, "XYGraph Ref"=w487) -> ("Error Out"=w489:errorcluster, "Message"=w480:string, "File Path(s)"=w481:path[], "# Plots Added"=w490:i32[])  [unwired: 3 in, 2 out]
          n185 = Add Array Elements(numeric array=w490) -> (sum=w478:i32)
          n186 = Equal?(x=w477, y=w478) -> (x = y?=w486:bool)
          n187 = case shown="True" w486 {
            tunnel: w489 -> [w497 w506]
            tunnel: [w497 w503] -> w488
            tunnel: w487 -> [_ w502]
            tunnel: w485 -> [w498 w501]
            tunnel: [w498 w500] -> w484
            tunnel: w483 -> [w496 w510]
            tunnel: [w496 w509] -> w482
            tunnel: w481 -> [_ _]
            tunnel: w480 -> [_ w508]
            tunnel: w479 -> [_ w499]
            frame False {
            }
            frame True {
              # "removes previous plot & updates data"
              n188 = Format Into String(format string="%s\n", initial string=w510, error in=w506, w508) -> (resulting string=w509:string, error out=w507:errorcluster)
              n189 = call "XY Graph Delete Plot.vi"("Error In"=w507, "Plot Index"=0, "XYGraph Ref"=w502) -> ("Error Out"=w504:errorcluster)  [unwired: 5 in, 3 out]
              n190 = call "Plot Editor_Plot to Data & Controls.vi"("Control Refnums"=w499, "XYGraph in"=w502, "error in (no error)"=w504, "Plot Editor Internal Data in"=w501) -> ("error out"=w503:errorcluster, "Plot Editor Internal Data out"=w500:T6)  [unwired: 6 in]
            }
          }
          n191 = call <vilib>:"Simple Error Handler.vi"("type of dialog (OK msg:1)"=w492, "error in (no error)"=w488) -> ("error out"=w493:errorcluster)  [unwired: 3 in, 4 out]
          n192 = call <vilib>:"Clear Errors.vi"("error in (no error)"=w493) -> ("error out"=w491:errorcluster)  [unwired: 5 in, 1 out]
        }
        frame "Delete out-of-bound Values" {
          n193 = call "Plot Editor_Remove out-of-bound Plot Values.vi"("Control Refnums"=w512, "XYGraph in"=w517, "error in (no error)"=w523, "Plot Editor Internal Data"=w514) -> ("error out"=w519:errorcluster, "Message"=w516:string, "Plot Editor Internal Data out"=w513:T6)  [unwired: 5 in]
          n194 = Format Into String(format string="%s\n", initial string=w522, error in=w519, w516) -> (resulting string=w521:string, error out=w518:errorcluster)
        }
        frame "Delete Element", Default {
          n195 = Variant To Data(error in=w528, type=cluster{"CtlRef":refnum<vi>, "Coords":T8} {"CtlRef"=refnum, "Coords"={"Horizontal"=0, "Vertical"=0}} ("output cluster"), Variant=w543) -> (data=w541:cluster{"CtlRef":refnum<vi>, "Coords":T8}, error out=w534:errorcluster)
          n196 = Unbundle(w541) -> ("CtlRef"=w540:refnum<vi>, "Coords"=w539:T8)
          n197 = call "Determine Clicked Array Element Index.vi"("Error In"=w534, "Coords of Click"=w539, "Array Refnum"=w540) -> ("Error Out"=w535:errorcluster, "Clicked Row"=w538:i32)  [unwired: 1 in, 6 out]
          n198 = case shown="0, Default" w538 {
            selector: w538 -> [w555 _]
            tunnel: w537 -> [w564 _]
            tunnel: w536 -> [w563 _]
            tunnel: w535 -> [w557 w566]
            tunnel: w533 -> [w559 w568]
            tunnel: [w558 w568] -> w532
            tunnel: w531 -> [w553 w567]
            tunnel: [w553 w567] -> w530
            tunnel: [w547 w566] -> w529
            tunnel: w527 -> [w551 w565]
            tunnel: w526 -> [w544 _]
            tunnel: w525 -> [w549 _]
            tunnel: [w550 w565] -> w524
            frame 0, Default {
              w560 = 1 ("length")
              n199 = property class="Arr (strict)"(reference=w564, error in=w557) -> (error out=w554:errorcluster, "Value"=w562:dbl[])  [unwired: 1 out]
              n200 = property class="Arr (strict)"(reference=w563, error in=w557) -> (error out=w552:errorcluster, "Value"=w561:dbl[])  [unwired: 1 out]
              n201 = Format Into String(format string="Deleted element %d\n", initial string=w559, error in=w557, w555) -> (resulting string=w558:string)  [unwired: 1 out]
              n202 = Delete From Array(array=w562, length=w560, index=w555) -> (array with subset deleted=w546:dbl[])  [unwired: 1 out]
              n203 = Delete From Array(array=w561, length=w560, index=w555) -> (array with subset deleted=w545:dbl[])  [unwired: 1 out]
              n204 = Merge Errors(w554, w552) -> (w548:errorcluster)
              n205 = call "Plot Editor_Data to Controls & Plot.vi"("Plot Editor Internal Data"=w551, "XYGraph in"=w549, "X Array"=w546, "Y Array"=w545, "error in (no error)"=w548, "Control Refnums"=w544) -> ("Plot Editor Internal Data"=w550:T6, "error out"=w547:errorcluster)  [unwired: 8 in]
            }
            frame -1 {
            }
          }
        }
        frame "Insert Element Before" {
          n206 = Variant To Data(error in=w574, type=cluster{"CtlRef":refnum<vi>, "Coords":T8} {"CtlRef"=refnum, "Coords"={"Horizontal"=0, "Vertical"=0}} ("output cluster"), Variant=w588) -> (data=w586:cluster{"CtlRef":refnum<vi>, "Coords":T8}, error out=w579:errorcluster)
          n207 = Unbundle(w586) -> ("CtlRef"=w585:refnum<vi>, "Coords"=w584:T8)
          n208 = call "Determine Clicked Array Element Index.vi"("Error In"=w579, "Coords of Click"=w584, "Array Refnum"=w585) -> ("Error Out"=w580:errorcluster, "Clicked Row"=w583:i32)  [unwired: 1 in, 6 out]
          n209 = case shown="0, Default" w583 {
            selector: w583 -> [w602 _]
            tunnel: w582 -> [w609 _]
            tunnel: w581 -> [w608 _]
            tunnel: w580 -> [w600 w611]
            tunnel: w578 -> [w604 w613]
            tunnel: [w601 w613] -> w577
            tunnel: w576 -> [w599 w612]
            tunnel: [w599 w612] -> w575
            tunnel: [w593 w611] -> w573
            tunnel: w572 -> [w596 w610]
            tunnel: [w594 w610] -> w571
            tunnel: w570 -> [w595 _]
            tunnel: w569 -> [w589 _]
            frame 0, Default {
              w605 = nan ("new element/subarray")
              n210 = property class="Arr (strict)"(reference=w609, error in=w600) -> (error out=w598:errorcluster, "Value"=w607:dbl[])  [unwired: 1 out]
              n211 = property class="Arr (strict)"(reference=w608, error in=w600) -> (error out=w597:errorcluster, "Value"=w606:dbl[])  [unwired: 1 out]
              n212 = Insert Into Array(array=w607, index=w602, new element=w605) -> (w591:dbl[])
              n213 = Insert Into Array(array=w606, index=w602, new element=w605) -> (w590:dbl[])
              n214 = Format Into String(format string="Element inserted before %d\n", initial string=w604, error in=w600, w602) -> (resulting string=w601:string)  [unwired: 1 out]
              n215 = Merge Errors(w598, w597) -> (w592:errorcluster)
              n216 = call "Plot Editor_Data to Controls & Plot.vi"("Plot Editor Internal Data"=w596, "XYGraph in"=w595, "X Array"=w591, "Y Array"=w590, "error in (no error)"=w592, "Control Refnums"=w589) -> ("Plot Editor Internal Data"=w594:T6, "error out"=w593:errorcluster)  [unwired: 8 in]
            }
            frame -1 {
            }
          }
        }
        frame "Insert Element After" {
          n217 = Variant To Data(error in=w619, type=cluster{"CtlRef":refnum<vi>, "Coords":T8} {"CtlRef"=refnum, "Coords"={"Horizontal"=0, "Vertical"=0}} ("output cluster"), Variant=w633) -> (data=w631:cluster{"CtlRef":refnum<vi>, "Coords":T8}, error out=w626:errorcluster)
          n218 = Unbundle(w631) -> ("CtlRef"=w628:refnum<vi>, "Coords"=w627:T8)
          n219 = call "Determine Clicked Array Element Index.vi"("Error In"=w626, "Coords of Click"=w627, "Array Refnum"=w628) -> ("Error Out"=w625:errorcluster, "Clicked Row"=w624:i32)  [unwired: 1 in, 6 out]
          n220 = case shown="0, Default" w624 {
            selector: w624 -> [w651 _]
            tunnel: w630 -> [w655 _]
            tunnel: w629 -> [w654 _]
            tunnel: w625 -> [w646 w657]
            tunnel: w623 -> [w649 w659]
            tunnel: [w647 w659] -> w622
            tunnel: w621 -> [w637 w658]
            tunnel: [w637 w658] -> w620
            tunnel: [w639 w657] -> w618
            tunnel: w617 -> [w644 w656]
            tunnel: [w638 w656] -> w616
            tunnel: w615 -> [w634 _]
            tunnel: w614 -> [w635 _]
            frame 0, Default {
              w650 = nan ("new element/subarray")
              n221 = property class="Arr (strict)"(reference=w655, error in=w646) -> (error out=w642:errorcluster, "Value"=w653:dbl[])  [unwired: 1 out]
              n222 = property class="Arr (strict)"(reference=w654, error in=w646) -> (error out=w641:errorcluster, "Value"=w652:dbl[])  [unwired: 1 out]
              n223 = Increment(x=w651) -> (x+1=w645:i32)
              n224 = Insert Into Array(array=w653, index=w645, new element=w650) -> (w643:dbl[])
              n225 = Format Into String(format string="Element inserted after %d\n", initial string=w649, error in=w646, w645) -> (resulting string=w647:string)  [unwired: 1 out]
              n226 = Insert Into Array(array=w652, index=w645, new element=w650) -> (w636:dbl[])
              n227 = Merge Errors(w642, w641) -> (w640:errorcluster)
              n228 = call "Plot Editor_Data to Controls & Plot.vi"("Plot Editor Internal Data"=w644, "XYGraph in"=w635, "X Array"=w643, "Y Array"=w636, "error in (no error)"=w640, "Control Refnums"=w634) -> ("Plot Editor Internal Data"=w638:T6, "error out"=w639:errorcluster)  [unwired: 8 in]
            }
            frame -1 {
            }
          }
        }
        frame "Update output string" {
          n229 = call-poly "Variant to Data.vi"("Variant"=w667) -> ("String"=w661:string)  [unwired: 8 in]
          n230 = Format Into String(format string="%s\n", initial string=w666, error in=w662, w661) -> (resulting string=w665:string, error out=w663:errorcluster)
        }
        frame "Delete NaN-containing Pairs" {
          n231 = call-poly "Variant to Data.vi"("Variant"=w684) -> ()  [unwired: 8 in, 1 out]
          n232 = Unbundle By Name(w672) -> ("X Array"=w683:dbl[], "Y Array"=w682:dbl[])
          n233 = call "Remove NaN-containing Pairs.vi"("Error In"=w678, "Y Array in"=w682, "X Array in"=w683) -> ("Error Out"=w677:errorcluster, "Y Array out"=w674:dbl[], "# X elts deleted"=w681:i32, "X Array out"=w675:dbl[])  [unwired: 5 in]
          n234 = case shown="1, Default" w681 {
            selector: w681 -> [_ w700]
            tunnel: [w687 w699] -> w679
            tunnel: w680 -> [w687 w697]
            tunnel: w677 -> [w686 w692]
            tunnel: [w686 w696] -> w676
            tunnel: w675 -> [_ w695]
            tunnel: w674 -> [_ w693]
            tunnel: w672 -> [w685 w694]
            tunnel: w671 -> [_ w691]
            tunnel: [w685 w690] -> w670
            tunnel: w669 -> [_ w689]
            frame 0 {
            }
            frame 1, Default {
              n235 = call "Plot Editor_Data to Controls & Plot.vi"("Plot Editor Internal Data"=w694, "XYGraph in"=w689, "X Array"=w695, "Y Array"=w693, "error in (no error)"=w692, "Control Refnums"=w691) -> ("Plot Editor Internal Data"=w690:T6, "error out"=w688:errorcluster)  [unwired: 8 in]
              n236 = Format Into String(format string="%d NaN-containing pair(s)  removed\n", initial string=w697, error in=w688, w700) -> (resulting string=w699:string, error out=w696:errorcluster)
            }
          }
        }
        frame "Fill Array with Ramp" {
          n237 = call-by-ref "?"("error in (no error)"=w711) -> ("error out"=w705:errorcluster, "OK?"=w710:bool, "Ramp"=w709:dbl[])  [unwired: 10 in, 2 out]
          n238 = case shown="True" w710 {
            tunnel: w713 -> [w717 w736]
            tunnel: [w717 w725] -> w712
            tunnel: w709 -> [_ w731]
            tunnel: w708 -> [w716 w735]
            tunnel: [w716 w734] -> w707
            tunnel: w706 -> [w715 w724]
            tunnel: w705 -> [w714 w723]
            tunnel: [w714 w720] -> w704
            tunnel: [w715 w724] -> w703
            tunnel: w702 -> [_ w719]
            tunnel: w701 -> [_ w718]
            frame False {
            }
            frame True {
              n239 = Array Size(array=w731) -> (size(s)=w730:i32)
              n240 = Decrement(x=w730) -> (x-1=w729:i32)
              n241 = Bundle By Name(cluster=w736, "X Array"=w731) -> (w727:T6)
              n242 = Index Array(array=w731, index #2=w729) -> (element #1=w732:dbl, element #2=w728:dbl)  [unwired: 1 in]
              n243 = call "Plot Editor_Store to Controls.vi"("Error In"=w723, "Control Refnums"=w719, "Plot Editor Internal Data in"=w727) -> ("Error Out"=w722:errorcluster, "Plot Editor Internal Data out"=w726:T6)  [unwired: 7 in]
              n244 = call "Plot Editor_Store to Plot.vi"("XYGraph in"=w718, "Error In"=w722, "Plot Editor Internal Data"=w726) -> ("Error Out"=w721:errorcluster, "Plot Editor Internal Data (dup)"=w725:T6)  [unwired: 7 in]
              n245 = Format Into String(format string="X array filled with ram (%#g...%#g [%d])\n", initial string=w735, error in=w721, w732, w728, w730) -> (resulting string=w734:string, error out=w720:errorcluster)
            }
          }
        }
        frame "Quit" {
          n246 = Unbundle By Name(w742) -> ("Original X Array"=w741:dbl[], "Original Y Array"=w740:dbl[], "Original XY Plot Properties"=w739:T2)
          n247 = Bundle By Name(cluster=w742, "X Array"=w741, "Y Array"=w740) -> (w743:T6)
        }
      }
      n248 = Empty Array?(array=w277) -> (empty?=w276:bool)
    }
    "Error" <- w239
  }
  "Plot Style out" <- w30
  "Error Out" <- w35
  n249 = Unregister For Events(event registration refnum=w25) -> ()  [unwired: 1 in, 1 out]
  n250 = Unbundle By Name(w34) -> ("Refnum based call"=w19:bool, "X Array"=w33:dbl[], "Y Array"=w32:dbl[])
  n251 = Release Queue(queue=w40) -> ()  [unwired: 2 in, 3 out]
  n252 = invoke class="VI" method="FP.Close"(reference=w20) -> (reference out=w17:refnum<vi>, error out=w13:errorcluster)  [unwired: 2 in, 1 out]
  n253 = case shown="False" w19 {
    tunnel: w17 -> [w746 w750]
    tunnel: [w746 w749] -> w16
    tunnel: [w745 w748] -> w14
    tunnel: w13 -> [w745 w747]
    frame False {
    }
    frame True {
      n254 = invoke class="VI" method="Abort VI"(reference=w750, error in=w747) -> (reference out=w749:refnum<vi>, error out=w748:errorcluster)  [unwired: 1 in, 1 out]
    }
  }
  n255 = Bundle("X Array"=w33, "Y Array"=w32) -> (→"Plot out":cluster{"X Array":dbl[], "Y Array":dbl[]})  [unwired: 1 in]
  n256 = Close Reference(reference=w16, error in (no error)=w14) -> (error out=w15:errorcluster)
  n257 = call "Clear Error.vi"("Error In"=w15) -> ()  [unwired: 8 in, 1 out]
